vi "Simultaneous Start.vi"() -> ()   [LabVIEW 2009]
uses:
  <vilib>/DAQmx/write.llb/DAQmx Write (Analog Wfm 1Chan NSamp).vi
  <vilib>/DAQmx/create/channels.llb/DAQmx Create Channel (AO-Voltage-Basic).vi
  <vilib>/DAQmx/create/channels.llb/DAQmx Create Channel (AI-Voltage-Basic).vi
  Program Files/National Instruments/LabVIEW 2009/resource/objmgr/daqmx.rc
  <vilib>/DAQmx/configure/timing.llb/DAQmx Timing (Sample Clock).vi
  <vilib>/measure/NI_MABase.lvlib
  <vilib>/DAQmx/read.llb/DAQmx Read (Analog 1D DBL 1Chan NSamp).vi
panel:
  out "data":dbl[](graph)
  out "signal out":waveform(dbl)(graph)
  in  "stop":bool
  in  "input rate":dbl=1000.0 format="%0.2f"
  in  "output rate":dbl(slide)=1000.0 scale=100.0..2000.0
  in  "AI channel":tag
  in  "AO channel":tag
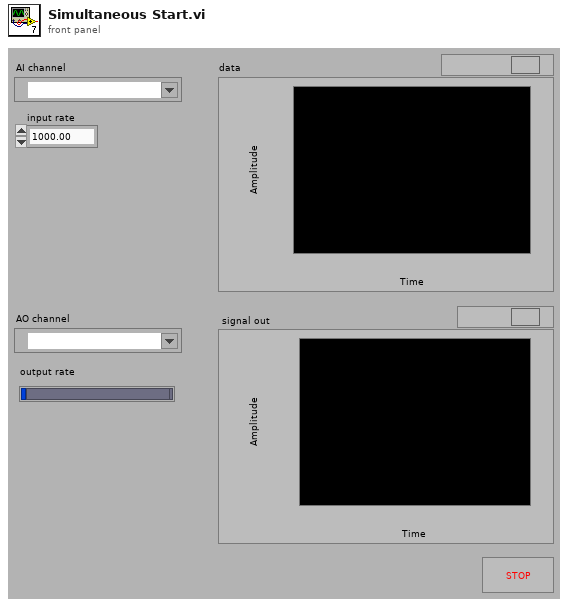
[diagram p1: front panel]
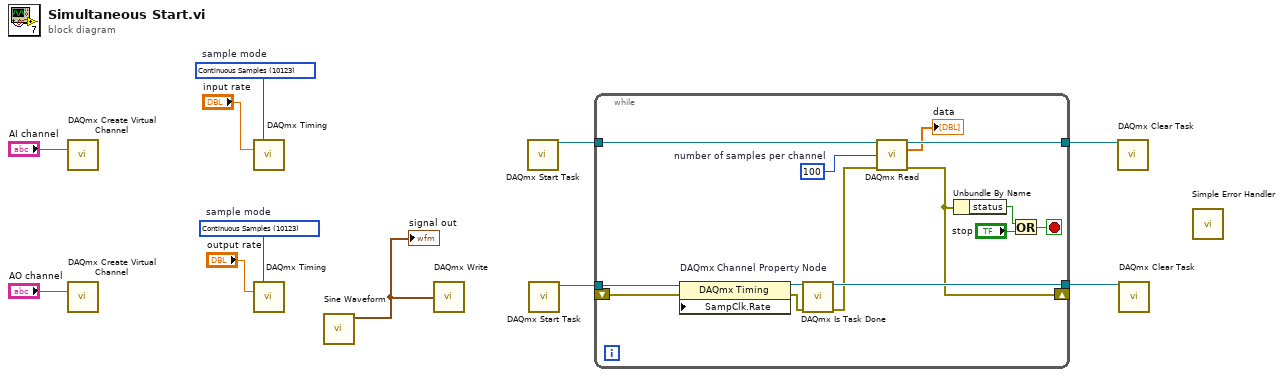
[diagram p0: block diagram]
diagram:
  w1 = 10123 items=["Finite Samples"=10178, "Continuous Samples"=10123, "Hardware Timed Single Point"=12522]  # sample mode
  w2 = 10123 items=["Finite Samples"=10178, "Continuous Samples"=10123, "Hardware Timed Single Point"=12522]  # sample mode
  n1 = call-poly <vilib>:"DAQmx Create Virtual Channel.vi"("physical channels"="AI channel") -> ()  [unwired: 13 in, 2 out]
  n2 = call-poly <vilib>:"DAQmx Create Virtual Channel.vi"("physical channels"="AO channel") -> ()  [unwired: 13 in, 2 out]
  n3 = call-poly <vilib>:"DAQmx Timing.vi"("sample mode"=w2, "rate"="input rate") -> ()  [unwired: 12 in, 2 out]
  n4 = call-poly <vilib>:"DAQmx Timing.vi"("sample mode"=w1, "rate"="output rate") -> ()  [unwired: 12 in, 2 out]
  n5 = call <vilib>:"Sine Waveform.vi"() -> ("signal out"=w3:waveform(dbl))  [unwired: 10 in, 1 out]
  "signal out" <- w3
  n6 = call-poly <vilib>:"DAQmx Write.vi"("data"=w3) -> ()  [unwired: 12 in, 3 out]
  n7 = call <vilib>:"DAQmx Start Task.vi"() -> ("task out"=w9:refnum<k21>)  [unwired: 14 in, 1 out]
  n8 = call <vilib>:"DAQmx Start Task.vi"() -> ("task out"=w10:refnum<k21>)  [unwired: 14 in, 1 out]
  n9 = while {
    tunnel: [w24] -> w11
    tunnel: w10 -> [w22]
    tunnel: w9 -> [w21]
    tunnel: [w20] -> w8
    shift-right: [w18] -> _
    shift-left: _ -> [w13]
    stop <- w15 stop-if-true
    w14 = 100  # number of samples per channel
    n10 = property on="DAQmx Channel Property Node" class="DAQmx Timing" props=["SampClk.Rate"](reference=w22, error in=w13) -> (reference out=w23:refnum<k21>, error out=w25:errorcluster)  [unwired: 1 in]
    n11 = call <vilib>:"DAQmx Is Task Done.vi"("task/channels in"=w23, "error in"=w25) -> ("task out"=w24:refnum<k21>, "error out"=w19:errorcluster)  [unwired: 11 in, 1 out]
    n12 = call-poly <vilib>:"DAQmx Read.vi"("task/channels in"=w21, "number of samples per channel"=w14, "error in"=w19) -> ("task out"=w20:refnum<k21>, "data"=→"data":dbl[], "error out"=w18:errorcluster)  [unwired: 10 in]
    n13 = Unbundle By Name "Unbundle By Name"(w18) -> ("status"=w17:bool)
    n14 = Or(x=w17, y="stop") -> (x .or. y?=w15:bool)
  }
  n15 = call <vilib>:"DAQmx Clear Task.vi"("task in"=w8) -> ()  [unwired: 14 in, 1 out]
  n16 = call <vilib>:"DAQmx Clear Task.vi"("task in"=w11) -> ()  [unwired: 14 in, 1 out]
  n17 = call <vilib>:"Simple Error Handler.vi"() -> ()  [unwired: 5 in, 5 out]
